vi "LabVIEW_Read Temperature.vi"(0 "PC Comms Port":refnum<visa-resource-name>="COM3", 11 "error in (no error)":errorcluster) -> (4 "PC Comms Port Out":refnum<visa-resource-name>="COM1", 6 "Air Temperature (°C)":dbl min=25.0 max=80.0 step=0.1, 15 "error out":errorcluster)   [LabVIEW 2010]
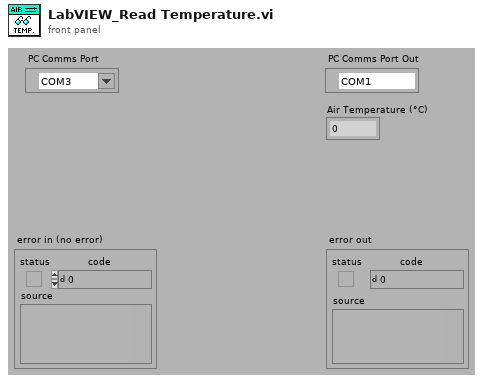
[diagram p1: front panel]
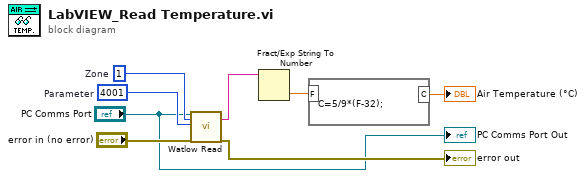
[diagram p0: block diagram]
diagram:
  w7 = u8 1  # Zone
  w8 = u32 4001  # Parameter
  n1 = call <instrlib>:"Watlow Read.vi"("PC Comms Port"="PC Comms Port", "Zone"=w7, "Parameter"=w8, "Error In"="error in (no error)") -> ("Read Value"=w4:string, "Error Out"=→"error out":errorcluster)  [unwired: 14 in]
  n2 = Fract/Exp String To Number(string=w4) -> (number=w6:dbl)  [unwired: 3 in, 1 out]
  n3 = formula code="C=5/9*(F-32);"("F"=w6) -> ("C"=→"Air Temperature (°C)":dbl)
  "PC Comms Port Out" <- "PC Comms Port"
